vi "UDPreciever2BinFile.vi"() -> ()   [LabVIEW 2012]
panel:
  out "length":i32
  out "built packet array":string[](array[string])
  out "channel":u32
  out "Raw Data Out":string
  out "error post-check":errorcluster
  out "End Reciever Error":errorcluster
  in  "stop reciever":bool
  out "port":u16
  out "error out post-read":errorcluster
  out "error out pre-read":errorcluster
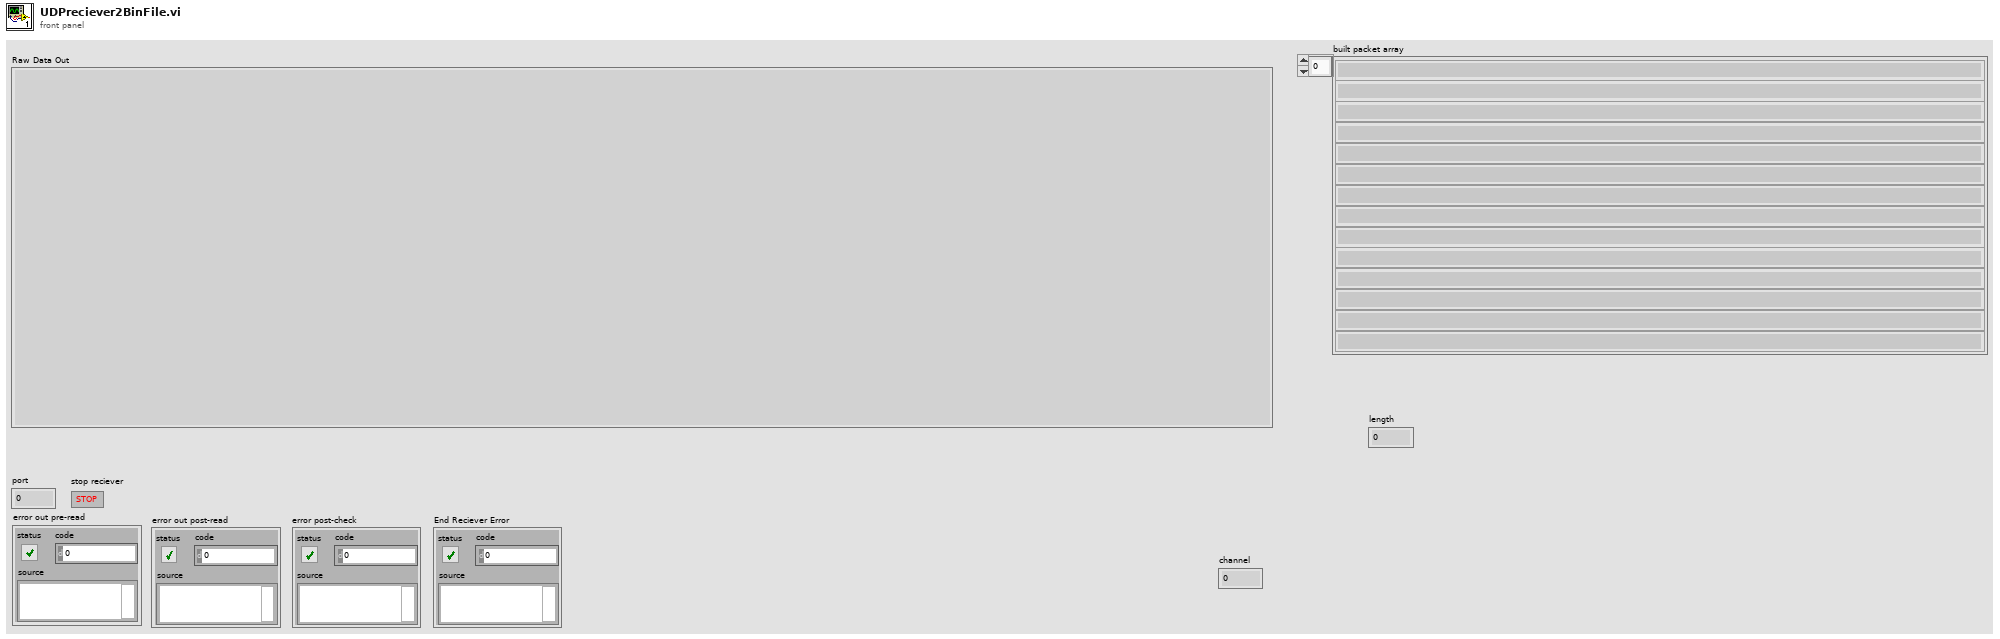
[diagram p1: front panel]
types:
  T1 = enum16{"open", "replace", "create", "open or create", "replace or create", "replace or create with confirmation"}
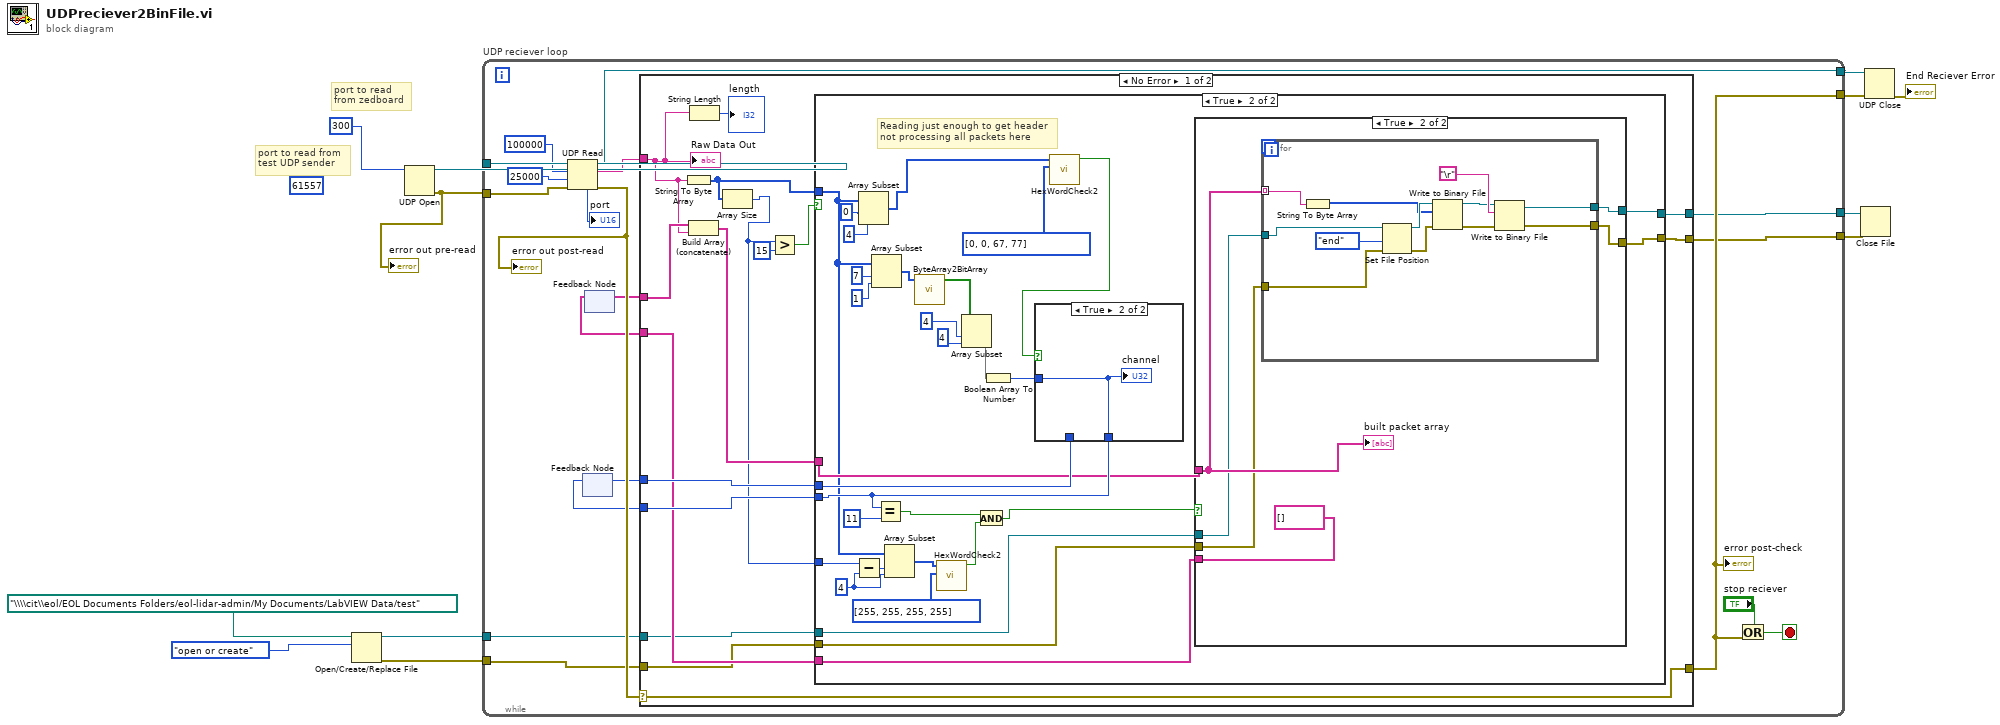
[diagram p0: block diagram]
diagram:
  (unwired) u16 61557 ("port")
  # "port to read \nfrom zedboard"
  # "port to read from \ntest UDP sender"
  n1 = Open/Create/Replace File(file path (use dialog)=path "\\\\cit\\eol/EOL Documents Folders/eol-lidar-admin/My Documents/LabVIEW Data/test" ("file (use dialog)"), operation (0:open)=T1."open or create") -> (refnum out=w4:refnum<file>, error out=w3:errorcluster)  [unwired: 4 in, 1 out]
  n2 = UDP Open(11:u16 300 ("port")) -> (port=w11:refnum<k16>, 0:w8:errorcluster)  [unwired: 4 in, 1 out]
  "error out pre-read" <- w8
  n3 = while "UDP reciever loop" {
    tunnel: [w31] -> w12
    tunnel: w11 -> [w30]
    tunnel: [w22] -> w10
    tunnel: w8 -> [w27]
    tunnel: w4 -> [w16]
    tunnel: w3 -> [w15]
    tunnel: [w14] -> w2
    tunnel: [w13] -> w1
    stop <- w29 stop-if-true
    n4 = UDP Read(connection ID=w30, max size (548)=100000, timeout ms (25000)=25000, 8:w27) -> (data out=w24:string, error out=w26:errorcluster, 3:w31:refnum<k16>, 4:→"port":u16)  [unwired: 1 out]
    "error out post-read" <- w26
    n5 = feedback #1() -> (w17:u32)  [unwired: 1 in]
    n6 = feedback #2() -> (w19:string[])  [unwired: 1 in]
    n7 = case shown="No Error" w26 {
      selector: w26 -> [w47 w110]
      tunnel: w24 -> [w33 _]
      tunnel: [w47 w110] -> w22
      tunnel: [w39 w109] -> w20
      tunnel: w19 -> [w46 w109]
      tunnel: [w43 w108] -> w18
      tunnel: w17 -> [w42 w108]
      tunnel: w16 -> [w37 w106]
      tunnel: w15 -> [w36 w107]
      tunnel: [w35 w106] -> w14
      tunnel: [w34 w107] -> w13
      frame No Error {
        n8 = String To Byte Array(string=w33) -> (unsigned byte array=w40:u8[])
        n9 = Build Array (concatenate)(w46, w33) -> (w41:string[])
        n10 = String Length(string=w33) -> (length=→"length":i32)
        n11 = Array Size(array=w40) -> (size(s)=w38:i32)
        n12 = Greater?(x=w38, y=15) -> (0:w45:bool)
        n13 = case shown="True" w45 {
          tunnel: w40 -> [_ w64]
          tunnel: [w51 w68] -> w43
          tunnel: w42 -> [w51 w69]
          tunnel: w38 -> [_ w72]
          tunnel: w41 -> [w50 w66]
          tunnel: [w50 w65] -> w39
          tunnel: w37 -> [w48 w55]
          tunnel: w36 -> [w49 w54]
          tunnel: [w48 w53] -> w35
          tunnel: [w49 w52] -> w34
          frame False {
          }
          frame True {
            w74 = 4 ("length")
            # "Reading just enough to get header\nnot processing all packets here"
            n14 = Subtract(x=w72, y=w74) -> (x-y=w73:i32)
            n15 = Array Subset(array=w64, index=0, length=4) -> (w78:u8[])
            n16 = Array Subset(array=w64, index=7, length=1) -> (w61:u8[])
            n17 = Array Subset(array=w64, index=w73, length=w74) -> (w67:u8[])
            n18 = call "ByteArray2BitArray.vi"("array"=w61) -> ("Array"=w58:bool[])  [unwired: 10 in]
            n19 = call "HexWordCheck2.vi"("array"=u8[] [255, 255, 255, 255], "Input Array"=w67) -> ("Boolean"=w75:bool)  [unwired: 9 in]
            n20 = Array Subset(array=w58, index=4, length=4) -> (w56:bool[])
            n21 = Boolean Array To Number(Boolean array=w56) -> (number=w57:u32)
            n22 = call "HexWordCheck2.vi"("array"=u8[] [0, 0, 67, 77], "Input Array"=w78) -> ("Boolean"=w79:bool)  [unwired: 9 in]
            n23 = case shown="True" w79 {
              tunnel: [w104 w105] -> w68
              tunnel: w69 -> [w104 _]
              tunnel: w57 -> [_ w105]
              frame False {
              }
              frame True {
                "channel" <- w105
              }
            }
            n24 = Equal?(x=w68, y=u32 11) -> (x = y?=w71:bool)
            n25 = And(x=w71, y=w75) -> (x .and. y?=w76:bool)
            n26 = case shown="True" w76 {
              tunnel: w66 -> [w85 w90]
              tunnel: [w85 string[] []] -> w65
              tunnel: w55 -> [w84 w89]
              tunnel: w54 -> [w83 w88]
              tunnel: [w84 w87] -> w53
              tunnel: [w83 w86] -> w52
              frame False {
              }
              frame True {
                n27 = for {
                  tunnel: w90 -> [w103] mode=indexing
                  tunnel: w89 -> [w101]
                  tunnel: w88 -> [w100]
                  tunnel: [w93] -> w87
                  tunnel: [w92] -> w86
                  n28 = String To Byte Array(string=w103) -> (unsigned byte array=w97:u8[])
                  n29 = Set File Position(refnum=w101, from (0:start)=enum16{"start", "end", "current"}."end", error in=w100) -> (refnum out=w99:refnum<file>, error out=w98:errorcluster)  [unwired: 1 in]
                  n30 = Write to Binary File(file (use dialog)=w99, data=w97, error in=w98) -> (refnum out=w95:refnum<file>, error out=w94:errorcluster)  [unwired: 3 in, 1 out]
                  n31 = Write to Binary File(file (use dialog)=w95, data="\r", error in=w94) -> (refnum out=w93:refnum<file>, error out=w92:errorcluster)  [unwired: 3 in, 1 out]
                }
                "built packet array" <- w90
              }
            }
          }
        }
        "Raw Data Out" <- w33
      }
      frame Error {
      }
    }
    "error post-check" <- w22
    n32 = feedback-in #1(w18) -> ()
    n33 = feedback-in #2(w20) -> ()
    n34 = Or(x="stop reciever", y=w22) -> (x .or. y?=w29:bool)
  }
  n35 = Close File(refnum=w2, error in=w1) -> ()  [unwired: 2 out]
  n36 = UDP Close(connection ID=w12, 8:w10) -> (error out=→"End Reciever Error":errorcluster)  [unwired: 1 out]
